vi "MF-101 Read Write TTL DIO.vi"() -> ()   [LabVIEW 8.6]
uses:
  vi.lib/UeiDaq/UeiDaqConfigureTimingForSimpleIO.vi
  vi.lib/UeiDaq/UeiDaqCreateDOSession.vi
  <libdir>/resource/objmgr/ueidaq.rc
  vi.lib/UeiDaq/UeiDaqCreateDISession.vi
  vi.lib/UeiDaq/UeiDaqReadOneDigitalScanUInt16.vi
  vi.lib/UeiDaq/UeiDaqWriteOneDigitalScanUInt16.vi
panel:
  out "TTY data":u16
  out "DO raw data decimal":u32[](array[numeric])
  in  "channels 2,3":u16(ring)
  in  "channels 0,1":u16(ring)
  out "Output Mask":u32[](array[numeric]) format="%04b"
  out "Total scans generated":u32
  out "device name":string
  out "DO Resolution (bits)":u32
  in  "Digital Output Resource":string
  in  "DO TTL Port":bool[][](array[boolean])
  out "DO raw data binary":u32[](array[numeric]) format="%b"
  out "current time":timestamp format="%<%X\n%x>T"
  out "device name":string
  out "DI Resolution (bits)":u32
  out "DI raw data":u16[](array[numeric]) format="%b"
  out "DI TTL Port":bool[][](array[boolean])
  in  "Digital Input Resource":string
  out "Total scans acquired":u32
  in  "Refresh rate (ms)":i32
  in  "stop":bool
  # "MF-101 READ WRITE TTL (Transistor-Transistor Logic) DIO Ports"
  # "1/ Set the resource name -->"
  # "2/ Set the update rate -->"
  # "3/ Set DIO direction -->"
  # "For TTL channels use resources:\n   pdna://192.168.100.2/dev0/do1/0\n   pdna://192.168.100.2/dev0/di1/0"
  # "For FET channels use resources:\n   pdna://192.168.100.2/dev0/do0\n   pdna://192.168.100.2/dev0/di0"
  # "with dongle ch 0,1 write - ch 2,3 read\n   ch0 on lights 0,2 - ch1 on lights 1,3\n\nwith dongle ch 0,1 read - ch 2,3 write\n   ch2 on lights 0,2 - ch3 on lights 1,3"
  # "channel"
  # "3"
  # "2"
  # "1"
  # "0"
  # "DI Device info"
  # "DO Device info"
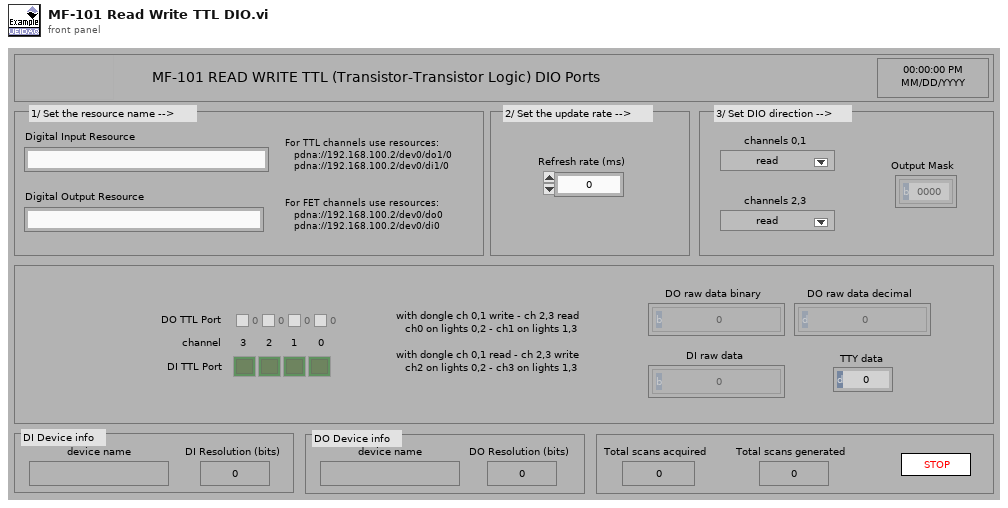
[diagram p1: front panel]
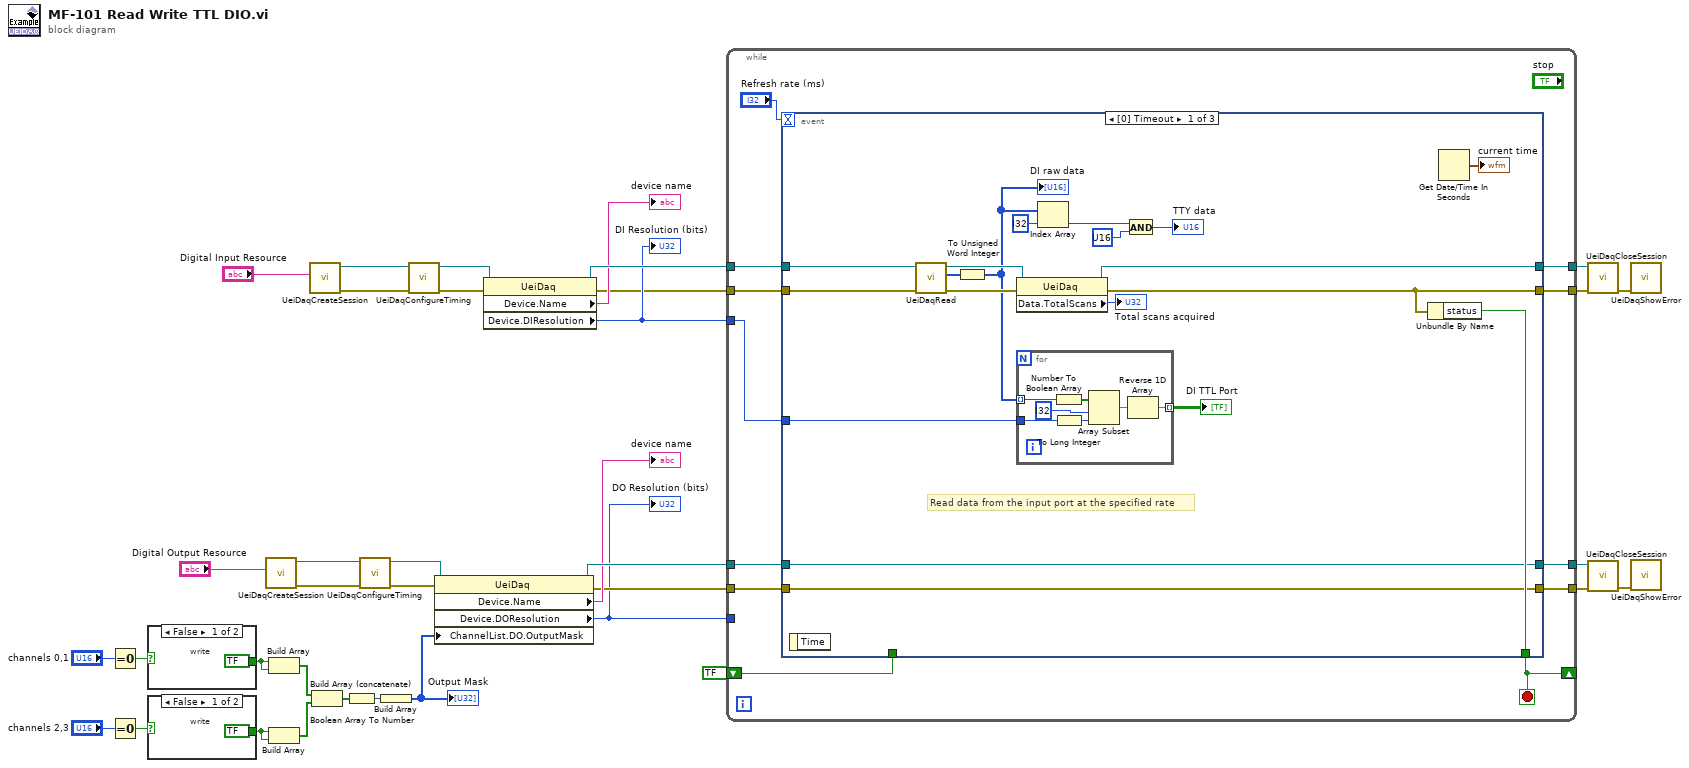
[diagram p0: block diagram]
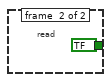
[diagram p2: hidden frame]
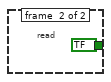
[diagram p3: hidden frame]
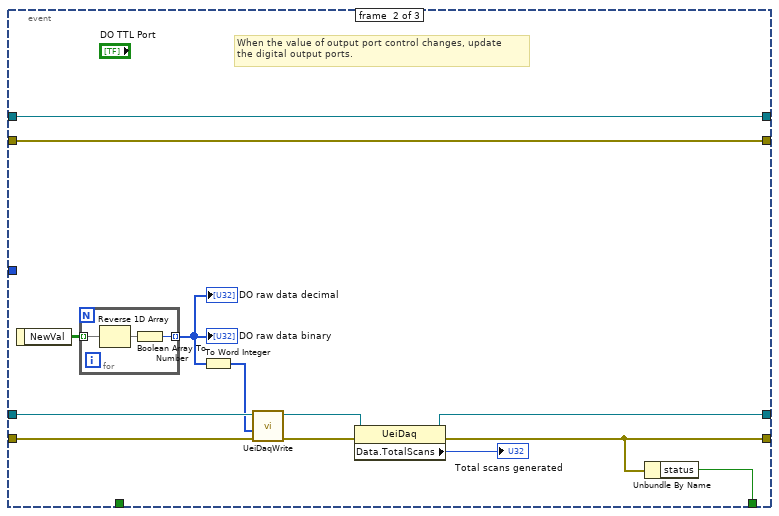
[diagram p4: hidden frame]
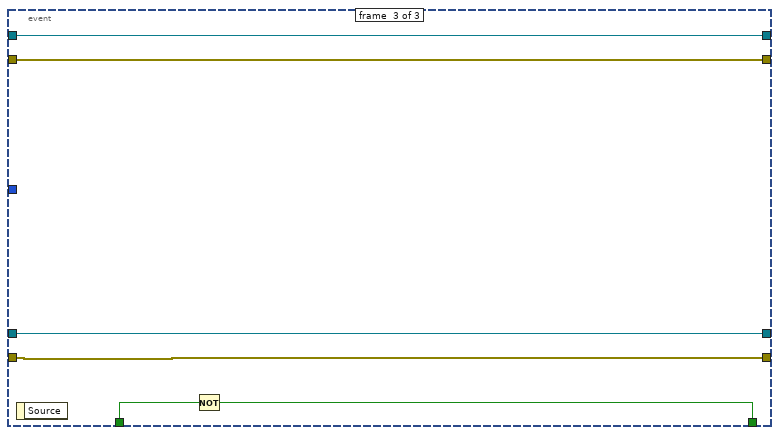
[diagram p5: hidden frame]
diagram:
  n1 = Equal To 0?(x="channels 0,1") -> (x = 0?=w10:bool)
  n2 = Equal To 0?(x="channels 2,3") -> (x = 0?=w7:bool)
  n3 = case shown="False" w10 {
    tunnel: [bool ? bool ?] -> w9
    frame #0 {
      # "write"
    }
    frame #1 {
      # "read"
    }
  }
  n4 = case shown="False" w7 {
    tunnel: [bool ? bool ?] -> w8
    frame #0 {
      # "write"
    }
    frame #1 {
      # "read"
    }
  }
  n5 = call-poly "UeiDaqCreateSession.vi"("Resource"="Digital Output Resource") -> ("error out"=w23:errorcluster, "UeiDaq Refnum Out"=w24:refnum<k20>)  [unwired: 3 in, 6 out]
  n6 = Build Array(w9, w9) -> (w5:bool[])
  n7 = Build Array(w8, w8) -> (w4:bool[])
  n8 = call-poly "UeiDaqCreateSession.vi"("Resource"="Digital Input Resource") -> ("error out"=w34:errorcluster, "UeiDaq Refnum Out"=w35:refnum<k20>)  [unwired: 2 in, 7 out]
  n9 = Build Array (concatenate)(w5, w4) -> (w3:bool[])
  n10 = Boolean Array To Number(Boolean array=w3) -> (number=w2:u32)
  n11 = call-poly "UeiDaqConfigureTiming.vi"("error in (no error)"=w23, "UeiDaq Refnum In"=w24) -> ("error out"=w20:errorcluster, "UeiDaq Refnum Out"=w21:refnum<k20>)  [unwired: 1 in, 7 out]
  n12 = Build Array(w2) -> (w1:u32[])
  "Output Mask" <- w1
  n13 = call-poly "UeiDaqConfigureTiming.vi"("error in (no error)"=w34, "UeiDaq Refnum In"=w35) -> ("error out"=w30:errorcluster, "UeiDaq Refnum Out"=w32:refnum<k20>)  [unwired: 1 in, 7 out]
  n14 = property class="UeiDaq"(reference=w21, error in=w20, "ChannelList.DO.OutputMask"=w1) -> (reference out=w19:refnum<k20>, error out=w14:errorcluster, "Device.Name"=→"device name":string, "Device.DOResolution"=w12:u32)
  "DO Resolution (bits)" <- w12
  n15 = property class="UeiDaq"(reference=w32, error in=w30) -> (reference out=w31:refnum<k20>, error out=w13:errorcluster, "Device.Name"=→"device name":string, "Device.DIResolution"=w27:u32)
  "DI Resolution (bits)" <- w27
  n16 = while {
    tunnel: w31 -> [w44]
    tunnel: w13 -> [w42]
    tunnel: [w43] -> w29
    tunnel: [w45] -> w28
    tunnel: w27 -> [w41]
    tunnel: w19 -> [w52]
    tunnel: w14 -> [w51]
    tunnel: [w50] -> w18
    tunnel: [w49] -> w17
    tunnel: w12 -> [_]
    shift-right: [w46] -> _
    shift-left: bool ? ("x") -> [w47]
    stop <- w46 stop-if-true
    n17 = event shown="[0] Timeout" {
      selector: _ -> [_ _ _]
      dyn-events: _ -> [_ _ _]
      timeout: "Refresh rate (ms)" -> [_ _ _]
      tunnel: [w63 w84 w99] -> w49
      tunnel: [w64 w88 w98] -> w50
      tunnel: [w65 w81 w100] -> w46
      tunnel: w52 -> [w64 w90 w98]
      tunnel: w51 -> [w63 w89 w99]
      tunnel: w47 -> [_ _ w97]
      tunnel: [w62 w83 w96] -> w45
      tunnel: w44 -> [w61 w83 w96]
      tunnel: [w60 w82 w95] -> w43
      tunnel: w42 -> [w59 w82 w95]
      tunnel: w41 -> [w58 _ _]
      event #0 {
        # "Read data from the input port at the specified rate"
        n18 = event-data() -> ()  [unwired: 2 out]
        n19 = call-poly "UeiDaqRead.vi"("error in (no error)"=w59, "UeiDaq Refnum In"=w61) -> ("error out"=w66:errorcluster, "Raw Data"=w69:i16[], "UeiDaq Refnum Out"=w67:refnum<k20>)  [unwired: 7 out]
        n20 = To Unsigned Word Integer(number=w69) -> (unsigned 16bit integer=w57:u16[])
        "DI raw data" <- w57
        n21 = property class="UeiDaq"(reference=w67, error in=w66) -> (reference out=w62:refnum<k20>, error out=w60:errorcluster, "Data.TotalScans"=→"Total scans acquired":u32)
        n22 = for {
          tunnel: w57 -> [w78] mode=indexing
          tunnel: w58 -> [w75]
          tunnel: [w73] -> w70 mode=indexing
          n23 = Number To Boolean Array(number=w78) -> (Boolean array=w77:bool[])
          n24 = To Long Integer(number=w75) -> (32bit integer=w72:i32)
          n25 = Array Subset(array=w77, index=i32 ?, length=w72) -> (w74:bool[])
          n26 = Reverse 1D Array(array=w74) -> (reversed array=w73:bool[])
        }
        "DI TTL Port" <- w70
        n27 = Index Array(array=w57, index=i32 ?) -> (element=w55:u16)
        n28 = And(x=w55, y=u16 ?) -> (x .and. y?=→"TTY data":u16)
        n29 = Unbundle By Name(w60) -> ("status"=w65:bool)
        n30 = Get Date/Time In Seconds() -> (seconds since 1Jan1904=→"current time":timestamp)
      }
      event #1 {
        # "When the value of output port control changes, update\nthe digital output ports."
        n31 = event-data() -> ("NewVal"=w91:bool[][])  [unwired: 1 out]
        n32 = for {
          tunnel: w91 -> [w93] mode=indexing
          tunnel: [w94] -> w79 mode=indexing
          n33 = Reverse 1D Array(array=w93) -> (reversed array=w92:bool[])
          n34 = Boolean Array To Number(Boolean array=w92) -> (number=w94:u32)
        }
        "DO raw data binary" <- w79
        "DO raw data decimal" <- w79
        n35 = To Word Integer(number=w79) -> (16bit integer=w80:i16[])
        n36 = call-poly "UeiDaqWrite.vi"("error in (no error)"=w89, "Digital Data"=w80, "UeiDaq Refnum In"=w90) -> ("error out"=w86:errorcluster, "UeiDaq Refnum Out"=w87:refnum<k20>)  [unwired: 7 out]
        n37 = property class="UeiDaq"(reference=w87, error in=w86) -> (reference out=w88:refnum<k20>, error out=w84:errorcluster, "Data.TotalScans"=→"Total scans generated":u32)
        n38 = Unbundle By Name(w84) -> ("status"=w81:bool)
      }
      event #2 {
        n39 = event-data() -> ()  [unwired: 2 out]
        n40 = Not(x=w97) -> (.not. x?=w100:bool)
      }
    }
  }
  n41 = call "UeiDaqCloseSession.vi"("error in (no error)"=w29, "UeiDaq Refnum In"=w28) -> ("error out"=w36:errorcluster)  [unwired: 1 in, 8 out]
  n42 = call "UeiDaqCloseSession.vi"("error in (no error)"=w17, "UeiDaq Refnum In"=w18) -> ("error out"=w25:errorcluster)  [unwired: 1 in, 8 out]
  n43 = call "UeiDaqShowError.vi"("error in (no error)"=w36) -> ()  [unwired: 2 in, 9 out]
  n44 = call "UeiDaqShowError.vi"("error in (no error)"=w25) -> ()  [unwired: 2 in, 9 out]
